vi "CSM - Wait and Send Message for Reply.vi"(0 "State":string="API State", 1 "Current Module (\"\" to Generate an ID)":string, 5 "Arguments (\"\")":string, 7 "Target Module":string="Target", 9 "Wait (5000ms)":i32=5000, 11 "Error In (No Error)":errorcluster, 12 "Response Timeout (-2 Using Global Settings)":i32=-2) -> (6 "Response":string="DoA", 10 "Waited (ms)":u32, 14 "Source CSM":string, 15 "error out":errorcluster)   [LabVIEW 2017, in "Communicable State Machine.lvlib"]
doc: "Sends a synchronous message to the CSM and waits for a reply before continuing code execution. If the CSM module does not exist, this VI waits for the specified timeout duration. The following errors may occur:\n- If the module does not exist at the time of sending and the wait times out, this VI returns a timeout error.\n- If the message is sent but no reply message is received within the timeout, this VI returns a \"CSM Timeout Error\".\n\n\n> [!NOTE] <b>Synchronous Message</b>\n>\n> A synchronous message is a type of message. After a CSM sends a synchronous message, it pauses state transitions and waits for the callee to complete message processing. Synchronous messages are described via `-@`. A call from one JKISM module to another via a synchronous message is called a synchronous call.\n>\n> <b>Errors occurring at the Caller</b>:\n> - If the input target module is `\"\"`, a `NO Target Error` is generated.\n> - If the input module does not exist, a `Target Error` is generated.\n> - If the input module exists but does not complete processing within the specified time, a `Timeout Error` is generated.\n>\n> <b>Caller waits for return</b>:\n> - If the caller is a CSM module, it stays in the Parse State the Queue++ VI.\n> - If it is an API call, it stays in the calling VI, such as the CSM - Send Message and Wait for Reply VI.\n>\n> <b>Return</b>:\n> - <b>If the caller is a CSM module</b>:\n> - Normally, it enters the `Response` state to handle the return.\n> - If an error occurs at the caller, it causes the CSM state machine to enter the `Error Handler` module to handle the error.\n> - If an error occurs at the callee, this information is still the result of the message. It is handled in the `Response` state and can be obtained from Additional Information.\n> - <b>If it is an API call</b>:\n> - The Response output is the return.\n> - Errors occurring at both the caller and callee are merged into the error cluster output.\n\n\n> [!NOTE] <b>CSM Synchronous Message Global Timeout</b>\n>\n> - When performing CSM inter-module communication or using the VI that sends synchronous messages, the default timeout is -2, which uses the globally configured timeout.\n> - The global timeout can be set to other positive values using the CSM - Set TMO of Sync-Reply VI to override the global setting.\n> - The global timeout only applies to synchronous calls. Asynchronous calls are unaffected.\n\n\n> [!NOTE] <b>CSM Message Target Module Description</b>\n>\n> In Normal Mode, the target module for a CSM message is the specified module name.\n> System-level modules start with a `.` in their name. The target module for a CSM message includes the `.` in the name. For example, if the requested module name is `.System`, the target module for the CSM message is `.System`.\n> In Worker Mode, the target module for a CSM message can only be the overall module name, not the node name. For example, if the requested module name is `Worker#`, the target module for the CSM message is `Worker`.\n> In Chain of Responsibility Mode, the target module for a CSM message can only be the overall module name, not the node name. For example, if the requested module name is `Chain$1`, the target module for the CSM message is `Chain`.\n> In Chain of Responsibility Mode, a message is routed directly based on handling capability and priority (smaller number = higher priority) and is not passed sequentially across nodes.\n\n\n-- <b>Controls</b> --\n- <b>Current Module (\"\" to Generate an ID)</b>: Name of the current module. If empty, a temporary ID is generated for debugging purposes to identify the location.\n- <b>State</b>: Message string.\n- <b>Arguments (\"\")</b>: Message arguments.\n- <b>Target Module</b>: CSM module name.\n- <b>Wait (5000ms)</b>: Timeout duration for waiting. The default is 5000 ms.\n- <b>Response Timeout (-2 Using Global Settings)</b>: Timeout for synchronous calls. The default is -2, which uses the global setting. You can set the global timeout using the CSM - Set TMO of Sync-Reply VI.\n\n-- <b>Indicators</b> --\n- <b>Response</b>: Returned response.\n- <b>Source CSM</b>: Name of the CSM module that sourced the returned response. In Worker Mode or Chain of Responsibility Mode, this returns the name of the node."
uses:
  Communicable State Machine.lvlib
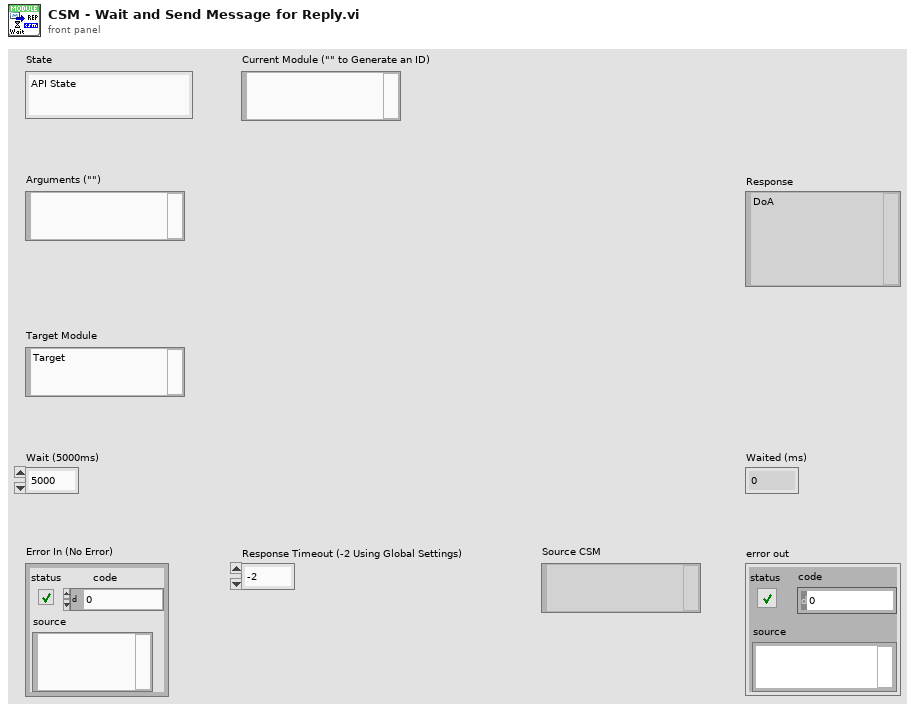
[diagram p1: front panel]
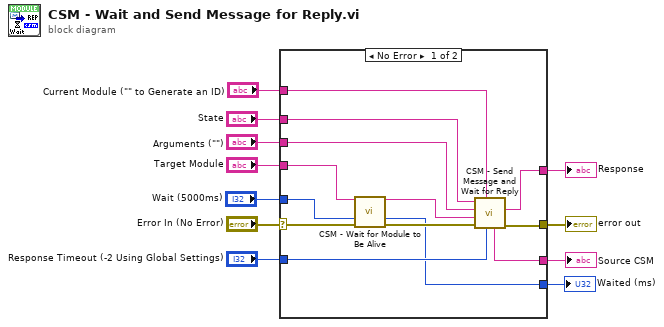
[diagram p0: block diagram]
diagram:
  n1 = case shown="No Error" "Error In (No Error)" {
    selector: "Error In (No Error)" -> [w24 w25]
    tunnel: "State" -> [w18 _]
    tunnel: "Response Timeout (-2 Using Global Settings)" -> [w13 _]
    tunnel: [w16 w25] -> w8
    tunnel: [w15 _] -> w7
    tunnel: "Target Module" -> [w23 _]
    tunnel: "Arguments (\"\")" -> [w19 _]
    tunnel: "Current Module (\"\" to Generate an ID)" -> [w17 _]
    tunnel: [w14 _] -> w3
    tunnel: "Wait (5000ms)" -> [w22 _]
    tunnel: [w12 _] -> w1
    frame No Error {
      n2 = call "CSM - Wait for Module to Be Alive.vi"("CSM Name"=w23, "Wait (5000 ms)"=w22, "error in (no error)"=w24) -> ("CSM Name (Dup)"=w20:string, "Waited (ms)"=w12:u32, "error out"=w21:errorcluster)  [unwired: 10 in]
      n3 = call "CSM - Send Message and Wait for Reply.vi"("Response Timeout (-2 Using Global Settings)"=w13, "Current Module (\"\" to Generate an ID)"=w17, "Error In (No Error)"=w21, "Target Module"=w20, "Arguments (\"\")"=w19, "State"=w18) -> ("error out"=w16:errorcluster, "Response"=w15:string, "Source CSM"=w14:string)  [unwired: 3 in]
    }
    frame Error {
    }
  }
  "error out" <- w8
  "Response" <- w7
  "Source CSM" <- w3
  "Waited (ms)" <- w1
